vi "CreateTriggerChannelCountNode.vi"(7 "DOM Document":refnum<k20>, 8 "Error In":errorcluster, 9 "Auto Count?":bool, 10 "Infinite?":bool, 11 "Count":u32) -> (0 "Error Out":errorcluster, 3 "Trigger Channel Count Node":refnum<k20>)   [LabVIEW 2012]
uses:
  libs/LV-Utilities/LV-Utilities.lvlib
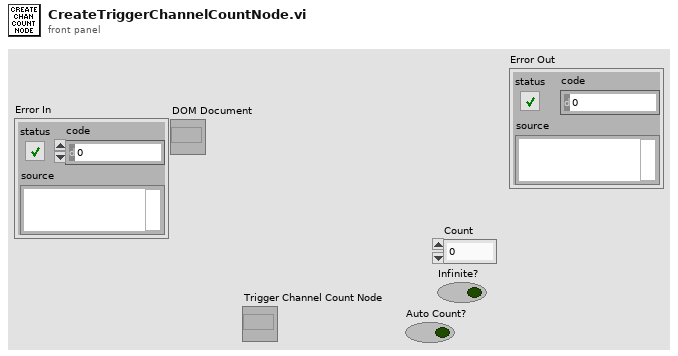
[diagram p1: front panel]
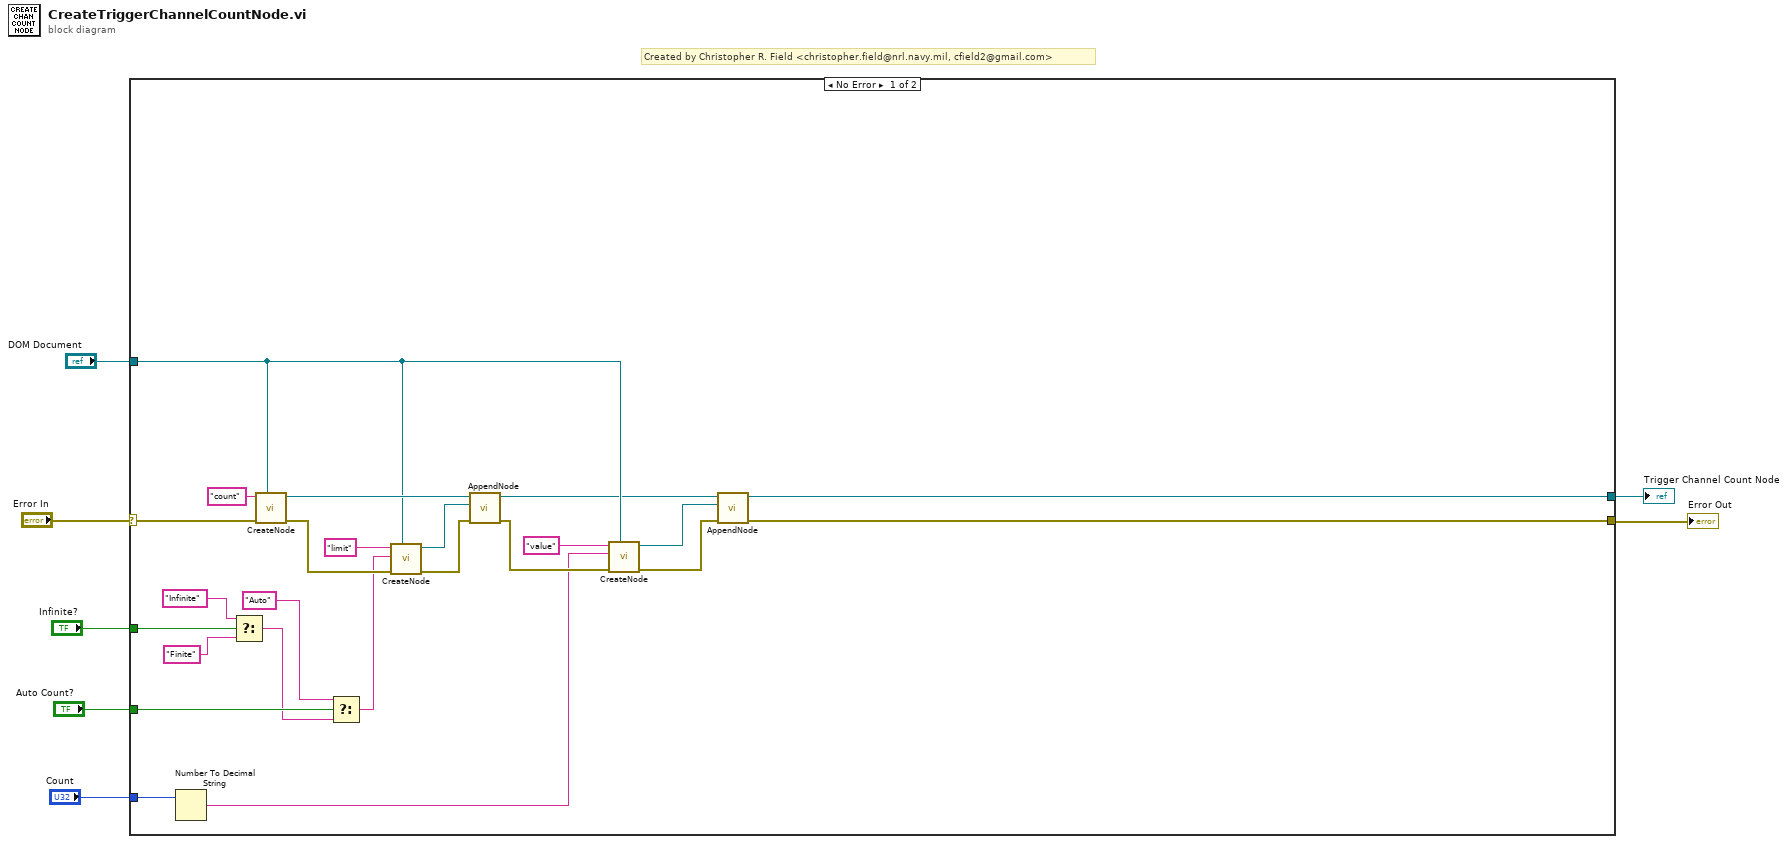
[diagram p0: block diagram]
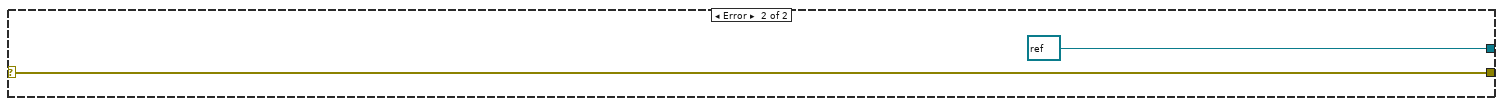
[diagram p2: hidden frame]
diagram:
  # "Created by Christopher R. Field <christopher.field@nrl.navy.mil, cfield2@gmail.com>"
  n1 = case shown="No Error" "Error In" {
    selector: "Error In" -> [w31 w33]
    tunnel: "DOM Document" -> [w18 _]
    tunnel: [w29 w33] -> w5
    tunnel: [w28 refnum<k20> refnum ("Wirings Node 2")] -> w4
    tunnel: "Count" -> [w24 _]
    tunnel: "Infinite?" -> [w23 _]
    tunnel: "Auto Count?" -> [w11 _]
    frame No Error {
      n2 = Number To Decimal String(number=w24) -> (decimal integer string=w16:string)  [unwired: 1 in]
      n3 = Select(t="Infinite", s=w23, f="Finite") -> (s? t:f=w10:string)
      n4 = call "CreateNode.vi"("DOM Document"=w18, "Error In"=w31, "Tag Name"="count") -> ("Error out"=w26:errorcluster, "Node"=w27:refnum<k20>)  [unwired: 7 in]
      n5 = Select(t="Auto", s=w11, f=w10) -> (s? t:f=w8:string)
      n6 = call "CreateNode.vi"("DOM Document"=w18, "Error In"=w26, "Text"=w8, "Tag Name"="limit") -> ("Error out"=w19:errorcluster, "Node"=w20:refnum<k20>)  [unwired: 6 in]
      n7 = call "AppendNode.vi"("Error In"=w19, "Child Node"=w20, "Parent Node In"=w27) -> ("Error Out"=w17:errorcluster, "Parent Node Out"=w14:refnum<k20>)  [unwired: 7 in]
      n8 = call "CreateNode.vi"("DOM Document"=w18, "Error In"=w17, "Text"=w16, "Tag Name"="value") -> ("Error out"=w13:errorcluster, "Node"=w12:refnum<k20>)  [unwired: 6 in]
      n9 = call "AppendNode.vi"("Error In"=w13, "Child Node"=w12, "Parent Node In"=w14) -> ("Error Out"=w29:errorcluster, "Parent Node Out"=w28:refnum<k20>)  [unwired: 7 in]
    }
    frame Error {
    }
  }
  "Trigger Channel Count Node" <- w4
  "Error Out" <- w5
